vi "Connection String.vi"(8 "error in (no error)":errorcluster, 11 "PostgreSQL in":refnum<class "PostgreSQL.lvclass">) -> (0 "error out":errorcluster, 2 "Connected String":string, 3 "PostgreSQL out":refnum<class "PostgreSQL.lvclass">)   [LabVIEW 2021, in "PostgreSQL.lvclass"]
uses:
  <userlib>/John_Lib/DataBase/PostgreSQL_API/PostgreSQL.lvclass
  <userlib>/John_Lib/DataBase/PostgreSQL_API/PostgreSQL.lvclass/PostgreSQL.ctl
  <userlib>/John_Lib/DataBase/NI_DB_API/NI_DB_API.lvclass
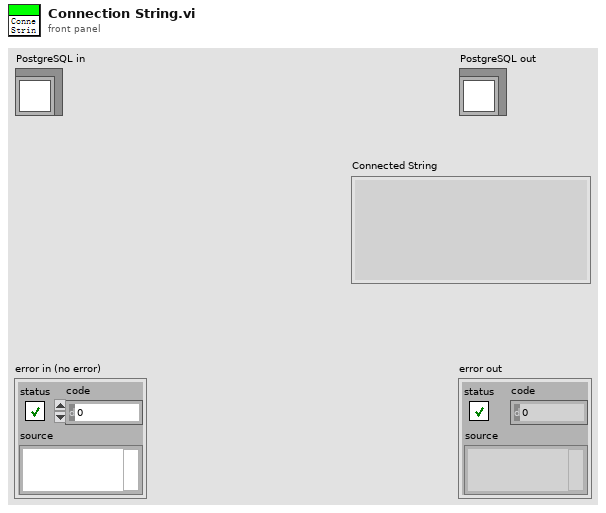
[diagram p1: front panel]
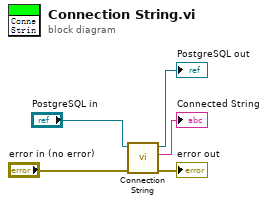
[diagram p0: block diagram]
diagram:
  n1 = call-parent "Connection String.vi"("error in (no error)"="error in (no error)", "DataBase_SQL in"="PostgreSQL in") -> ("error out"=→"error out":errorcluster, "Connected String"=→"Connected String":string, "DataBase_SQL out"=→"PostgreSQL out":refnum<class "PostgreSQL.lvclass">)  [unwired: 7 in]
